vi "Response Data to ListBox Row.vi"(8 "error in (no error)":errorcluster, 11 "Text based Communications Test in":refnum<class "Text based Communications Test.lvclass">) -> (0 "error out":errorcluster, 3 "Text based Communications Test out":refnum<class "Text based Communications Test.lvclass">)   [LabVIEW 2017, in "Text based Communications Test.lvlib" / "Text based Communications Test.lvclass"]
uses:
  Text based Communications Test.lvclass
  Text based Communications Test.lvclass/Text based Communications Test.ctl
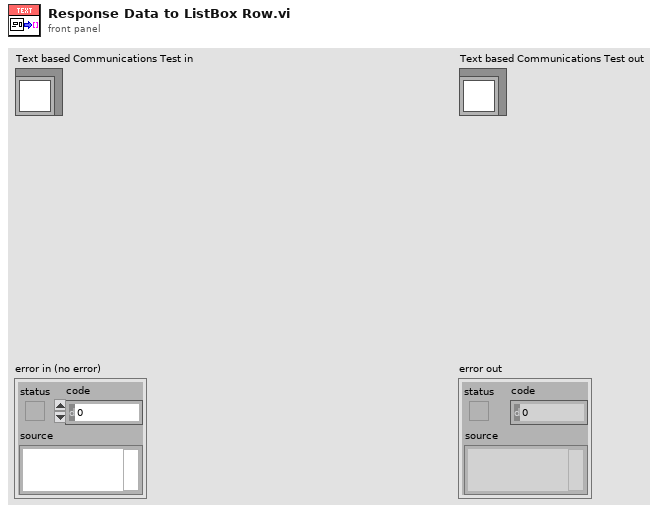
[diagram p1: front panel]
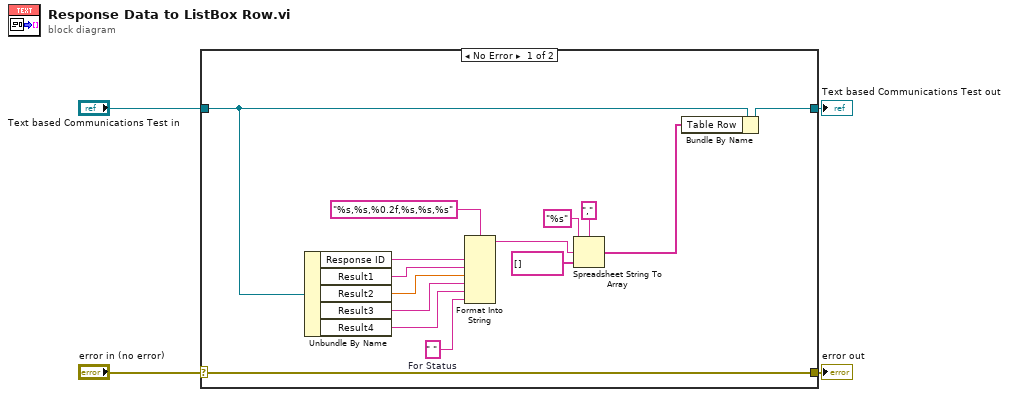
[diagram p0: block diagram]
diagram:
  n1 = case shown="No Error" "error in (no error)" {
    selector: "error in (no error)" -> [w19 w21]
    tunnel: [w19 w21] -> w3
    tunnel: [w9 w20] -> w1
    tunnel: "Text based Communications Test in" -> [w10 w20]
    frame No Error {
      w5 = " "  # For Status
      n2 = Unbundle By Name(w10) -> ("Response ID"=w17:string, "Result1"=w16:string, "Result2"=w15:dbl, "Result3"=w14:string, "Result4"=w13:string)
      n3 = Format Into String(format string="%s,%s,%0.2f,%s,%s,%s", w17, w16, w15, w14, w13, w5) -> (resulting string=w7:string)  [unwired: 2 in, 1 out]
      n4 = Spreadsheet String To Array(delimiter (Tab)=",", format string="%s", spreadsheet string=w7, array type (2D Dbl)=string[] []) -> (array=w8:string[])
      n5 = Bundle By Name(cluster=w10, "Table Row"=w8) -> (w9:refnum<class "Text based Communications Test.lvclass">)
    }
    frame Error {
    }
  }
  "error out" <- w3
  "Text based Communications Test out" <- w1
